vi "JSON Tree to LabVIEW Type.vi"(8 "error in (no error)":errorcluster, 10 "Ctl Refnum":refnum<vi>, 11 "JSON Tree In":variant) -> (0 "error out":errorcluster, 3 "JSON Tree Passthrough":variant)   [LabVIEW 2015, in "i3-json.lvlib"]
uses:
  i3-json.lvlib
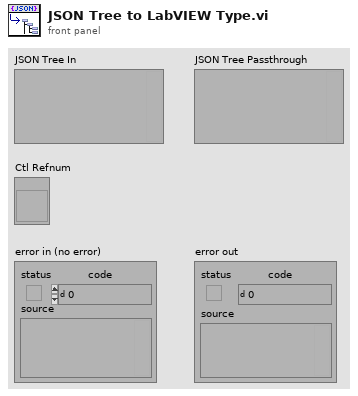
[diagram p1: front panel]
types:
  T1 = typedef "NI_Data Type.lvlib/Data Type.ctl" = enum8{"Invalid Type", "Void", "I8", "I16", "I32", "I64", "U8", "U16", "U32", "U64", "Single Float", "Double Float", "Extended Float", "Single Complex", "Double Complex", "Extended Complex", "Enum U8", "Enum U16", "Enum U32", "Enum U64", "Single Float With Unit", "Double Float With Unit", "Extended Float With Unit", "Single Complex with Unit", "Double Complex with Unit", "Extended Complex with Unit", "Boolean", "String", "Path", "Picture", "Tag", "Array", "Cluster", "Variant", "LV Variant", "Waveform", "Timestamp", "Digital Waveform", "Digital Data", "ExpressData", "Refnum", "External Data", "VI", "Poly VI", "LabVIEW Class Instance", "Fixed Point"}
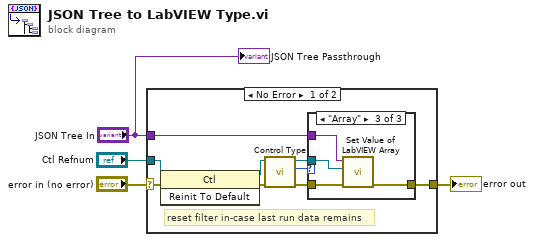
[diagram p0: block diagram]
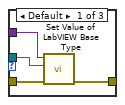
[diagram p2: hidden frame]
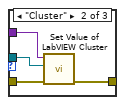
[diagram p3: hidden frame]
diagram:
  n1 = case shown="No Error" "error in (no error)" {
    selector: "error in (no error)" -> [w8 w26]
    tunnel: "Ctl Refnum" -> [w5 _]
    tunnel: [w10 w26] -> w2
    tunnel: "JSON Tree In" -> [w9 _]
    frame No Error {
      # "reset filter in-case last run data remains"
      n2 = invoke class="Ctl" method="Reinit To Default"(reference=w5, error in=w8) -> (reference out=w6:refnum<vi>, error out=w7:errorcluster)  [unwired: 1 in, 1 out]
      n3 = call "Control Type.vi"("error in (no error)"=w7, "Control in"=w6) -> ("error out"=w11:errorcluster, "Type"=w13:T1, "Control out"=w12:refnum<vi>)  [unwired: 7 in]
      n4 = case shown="\"Array\"" w13 {
        tunnel: w12 -> [w15 w19 w23]
        tunnel: w11 -> [w17 w20 w24]
        tunnel: w9 -> [w14 w18 w22]
        tunnel: [w16 w21 w25] -> w10
        frame Default {
          n5 = call "Set Value of LabVIEW Base Type.vi"("error in (no error)"=w17, "LabVIEW Base Type"=w15, "JSON Tree Node"=w14) -> ("error out"=w16:errorcluster)  [unwired: 8 in]
        }
        frame "Cluster" {
          n6 = call "Set Value of LabVIEW Cluster.vi"("error in (no error)"=w20, "LabVIEW Cluster"=w19, "JSON Tree Object"=w18) -> ("error out"=w21:errorcluster)  [unwired: 8 in]
        }
        frame "Array" {
          n7 = call "Set Value of LabVIEW Array.vi"("error in (no error)"=w24, "LabVIEW Array"=w23, "JSON Tree Array"=w22) -> ("error out"=w25:errorcluster)  [unwired: 8 in]
        }
      }
    }
    frame Error {
    }
  }
  "error out" <- w2
  "JSON Tree Passthrough" <- "JSON Tree In"
